vi "Autonomous Independent.vi"   [LabVIEW 2011]
doc: "This VI is called when autonomous begins, and will automatically be terminated when autonomous ends. You can carry out timed or sensor driven robot movement independently without needing to return to the caller."
uses:
  Robot Global Data.vi
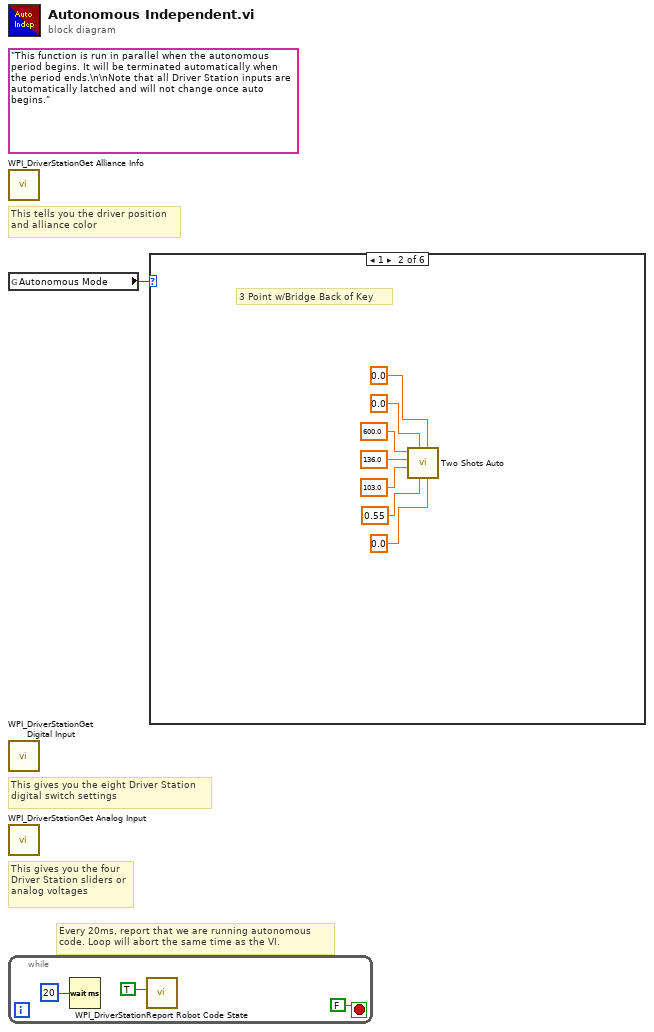
[diagram p0: block diagram]
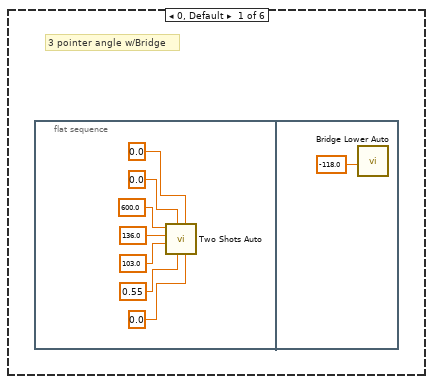
[diagram p2: hidden frame]
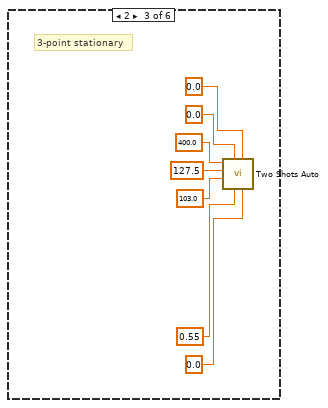
[diagram p3: hidden frame]
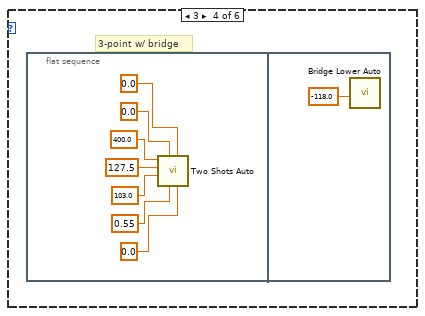
[diagram p4: hidden frame]
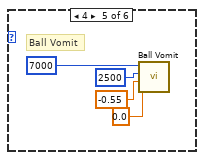
[diagram p5: hidden frame]
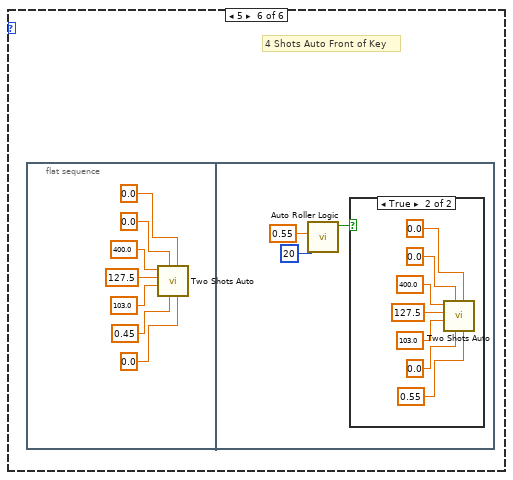
[diagram p6: hidden frame]
diagram:
  (unwired) "This function is run in parallel when the autonomous period begins. It will be terminated automatically when the period ends.\n\nNote that all Driver Station inputs are automatically latched and will not change once auto begins."
  # "Every 20ms, report that we are running autonomous\ncode. Loop will abort the same time as the VI."
  # "This tells you the driver position\nand alliance color"
  # "This gives you the eight Driver Station\ndigital switch settings"
  # "This gives you the four\nDriver Station sliders or\nanalog voltages"
  n1 = call <vilib>:"WPI_DriverStationGet Alliance Info.vi"() -> ()  [unwired: 12 out]
  n2 = global read "Robot Global Data.vi" "Autonomous Mode"() -> (w1:i16)
  n3 = call <vilib>:"WPI_DriverStationGet Digital Input.vi"() -> ()  [unwired: 12 out]
  n4 = call <vilib>:"WPI_DriverStationGet Analog Input.vi"() -> ()  [unwired: 12 out]
  n5 = while {
    stop <- FALSE stop-if-true
    n6 = Wait (ms)(milliseconds to wait=u32 20) -> ()  [unwired: 1 out]
    n7 = call <vilib>:"WPI_DriverStationReport Robot Code State.vi"("Autonomous"=TRUE) -> ()  [unwired: 10 in, 1 out]
  }
  n8 = case shown="1" w1 {
    frame 0, Default {
      # "3 pointer angle w/Bridge"
      n9 = flat-sequence {
        frame #0 {
          n10 = call "Two Shots Auto.vi"("chambering speed (back)"=0.0, "d trim"=0.0, "chambering speed (front)"=0.55, "h trim"=0.0, "Height"=103.0 ("Distance"), "Distance"=136.0 ("Height"), "backspin"=600.0) -> ()  [unwired: 5 in]
        }
        frame #1 {
          n11 = call "Bridge Lower Auto.vi"("d"=-118.0) -> ()  [unwired: 11 in]
        }
      }
    }
    frame 1 {
      # "3 Point w/Bridge Back of Key"
      n12 = call "Two Shots Auto.vi"("chambering speed (back)"=0.0, "d trim"=0.0, "chambering speed (front)"=0.55, "h trim"=0.0, "Height"=103.0 ("Distance"), "Distance"=136.0 ("Height"), "backspin"=600.0) -> ()  [unwired: 5 in]
    }
    frame 2 {
      # "3-point stationary"
      n13 = call "Two Shots Auto.vi"("chambering speed (back)"=0.0, "d trim"=0.0, "chambering speed (front)"=0.55, "h trim"=0.0, "Height"=103.0 ("Distance"), "Distance"=127.5 ("Height"), "backspin"=400.0) -> ()  [unwired: 5 in]
    }
    frame 3 {
      # "3-point w/ bridge"
      n14 = flat-sequence {
        frame #0 {
          n15 = call "Two Shots Auto.vi"("chambering speed (back)"=0.0, "d trim"=0.0, "chambering speed (front)"=0.55, "h trim"=0.0, "Height"=103.0 ("Distance"), "Distance"=127.5 ("Height"), "backspin"=400.0) -> ()  [unwired: 5 in]
        }
        frame #1 {
          n16 = call "Bridge Lower Auto.vi"("d"=-118.0) -> ()  [unwired: 11 in]
        }
      }
    }
    frame 4 {
      # "Ball Vomit"
      n17 = call "Ball Vomit.vi"("Rear Roller Speed"=0.0, "Front Roller Speed"=-0.55, "Roller Time"=u32 2500, "Wait Time(ms)"=u32 7000 ("Wait Time (ms)")) -> ()  [unwired: 8 in]
    }
    frame 5 {
      # "4 Shots Auto Front of Key"
      n18 = flat-sequence {
        frame #0 {
          n19 = call "Two Shots Auto.vi"("chambering speed (back)"=0.0, "d trim"=0.0, "chambering speed (front)"=0.45, "h trim"=0.0, "Height"=103.0 ("Distance"), "Distance"=127.5 ("Height"), "backspin"=400.0) -> ()  [unwired: 5 in]
        }
        frame #1 {
          n20 = call "Auto Roller Logic.vi"("Delay (ms)"=u32 20, "chambering speed"=0.55) -> ("ok"=w47:bool)  [unwired: 9 in]
          n21 = case shown="True" w47 {
            frame False {
            }
            frame True {
              n22 = call "Two Shots Auto.vi"("chambering speed (back)"=0.55, "d trim"=0.0, "chambering speed (front)"=0.0, "h trim"=0.0, "Height"=103.0 ("Distance"), "Distance"=127.5 ("Height"), "backspin"=400.0) -> ()  [unwired: 5 in]
            }
          }
        }
      }
    }
  }
